vi "MFLI read data.vi"(6 "Module":T3, 7 "ModuleHandles in":T5[](array[typedef]) {"ModHandle" format="0x%08x"; "Conn" format="0x%08x"}, 8 "error in (no error)":errorcluster, 9 "lock-in handle in":T1 {"Handle" format="0x%08x"; "Conn" format="0x%08x"}, 10 "Mode":T2, 11 "Queue in":T4) -> (2 "ModuleHandles out":T5[](array[typedef]) {"ModHandle" format="0x%08x"; "Conn" format="0x%08x"}, 3 "Handle Out out":T1 {"Handle" format="0x%08x"; "Conn" format="0x%08x"})   [LabVIEW 2024, in "Lock-in module.lvlib"]
uses:
  Lock-in module.lvlib
  <instrlib>/Zurich Instruments LabOne/Public/Modules/ziTypeModHandle.ctl
  Messenger service/Data types/Mailbox address.ctl
  Messenger service/Data types/Module name.ctl
  <instrlib>/Zurich Instruments LabOne/Public/ziTypeHandle.ctl
  ctl/Mode.ctl
  <instrlib>/Zurich Instruments LabOne/Public/Modules/ziTypeModEnum.ctl
  ctl/ADQ data.ctl
  <instrlib>/Zurich Instruments LabOne/Public/Configure/ziGetValueDemodSampleEx.vi
  <instrlib>/Zurich Instruments LabOne/Public/Modules/ziModGetScopeWave.vi
  <instrlib>/Zurich Instruments LabOne/Zurich Instruments LabOne.lvlib
  Messenger service/MessengerLib.lvlib
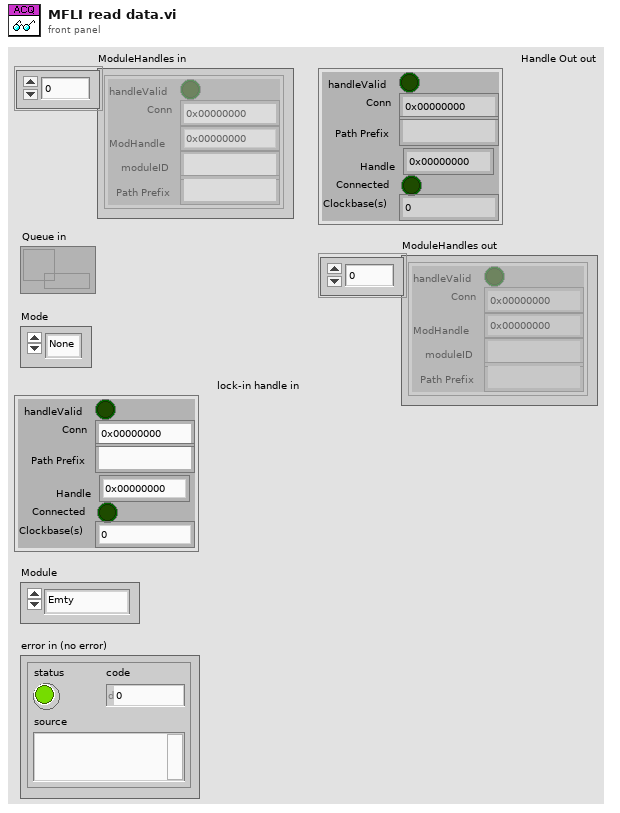
[diagram p1: front panel]
types:
  T1 = typedef "Zurich Instruments LabOne.lvlib/ziTypeHandle.ctl" = cluster{"handleValid":bool, "Conn":u64, "Path Prefix":string, "Handle":u64, "Connected":bool, "Clockbase(s)":dbl}
  T2 = typedef "Lock-in module.lvlib/Mode.ctl" = enum16{"None", "Point", "Scope", "Both", "DAQ"}
  T3 = typedef "Module name.ctl" = enum16{"Emty", "Magnet", "VTI", "Excitation", "Servo", "Acquisition", "Rotator", "Digitizer", "SMU2450", "Carousel", "Multimeter", "Tmp monitor", "Power monitor"}
  T4 = typedef "MessengerLib.lvlib/Mailbox address.ctl" = refnum<queue>
  T5 = typedef "Zurich Instruments LabOne.lvlib/ziTypeModHandle.ctl" = cluster{"handleValid":bool, "Conn":u64, "ModHandle":u64, "moduleID":string, "Path Prefix":string}
  T6 = typedef "Lock-in module.lvlib/ADQ data.ctl" = cluster{"X":sgl[], "Y":sgl[]}
  T7 = typedef "Zurich Instruments LabOne.lvlib/ziTypeDemodSampleSingle.ctl" = cluster{"Timestamps (ticks)":u64, "X (Vrms)":dbl, "Y (Vrms)":dbl, "Osc Phase (deg)":dbl, "Freq (Hz)":dbl, "DIO":u32, "AuxIn0 (V)":dbl, "AuxIn1 (V)":dbl, "Trigger":u32}
  T8 = typedef "Zurich Instruments LabOne.lvlib/ziTypeModEnum.ctl" = u16
  T9 = typedef "Zurich Instruments LabOne.lvlib/ziTypeModResults.ctl" = cluster{"PathArray":string[], "ValueType":T10, "NoOfResults":u64, "ziGenericHeader":T11[]}
  T10 = typedef "Zurich Instruments LabOne.lvlib/ziTypePollType.ctl" = enum16{"NONE", "DOUBLE_DATA", "INTEGER_DATA", "DEMOD_SAMPLE", "SCOPE_WAVE_HF2", "AUXIN_SAMPLE", "DIO_SAMPLE", "BYTE_ARRAY", "PWA_WAVE", "9", "10", "11", "12", "13", "14", "15", "TREE_CHANGE_DEPRI", "17", "ERROR", "19", "20", "21", "22", "23", "24", "25", "26", "27", "28", "29", "30", "31", "DOUBLE_DATA_TS", "INTEGER_DATA_TS", "34", "SCOPE_WAVE", "SCOPE_WAVE_EX", "37", "BYTE_ARRAY_TS", "39", "40", "41", "42", "43", "44", "45", "CNT_DATA", "47", "TREE_CHANGE", "49", "50", "51", "52", "53", "54", "55", "56", "57", "58", "59", "60", "61", "62", "63", "SWEEPER_DATA", "SPECTRUM_DATA", "ADVISOR_DATA", "VECTOR_DATA", "IMP_DATA"}
  T11 = typedef "Zurich Instruments LabOne.lvlib/ziTypeModGenericHeader.ctl" = cluster{"HeaderType":enum8{"HEADER_TYPE_NONE", "HEADER_TYPE_SWTRIGGER", "HEADER_TYPE_SWEEPER"}, "SampleFormat":u8, "SystemTime":timestamp, "CreatedTimeStamp":u64, "ChangedTimeStamp":u64, "Flags":u32, "ChunkSizeBytes":u64, "Name":string, "Status":u32, "GroupIndex":u32, "Color":u32, "ActiveRow":u32, "TriggerNumber":u64, "GridRows":u32, "GridCols":u32, "GridMode":u32, "GridOperation":u32, "GridDirection":u32, "GridRepetitions":u32, "GridColDelta":dbl, "GridColOffset":dbl, "GridRowDelta":dbl, "GridRowOffset":dbl, "Bandwidth":dbl, "Center":dbl, "Nenbw":dbl}
  T12 = typedef "Zurich Instruments LabOne.lvlib/ziTypeScopeWave.ctl" = cluster{"Timestamp (ticks)":u64, "Timestamp Trigger (ticks)":u64, "dt (s)":dbl, "Channel Enable":u8[], "Channel Input":enum8{"Signal Input 1", "Signal Input 2", "Trigger Input 1", "Trigger Input 2", "Aux Output 1", "Aux Output 2", "Aux Output 3", "Aux Output 4", "Aux Input 1", "Aux Input 2"}[], "Trigger Enable":u64, "Trigger Input":u64, "Channel BW Limit":u8[], "Channel Math":u8[], "Channel Scaling":sgl[], "Sequence Number":u32, "Segment Number":u32, "Block Number":u32, "Data Transfer Mode":enum8{"Single Transfer", "Block Transfer", "Continuous Transfer", "FFT Single Transfer"}, "Block Marker":enum8{"None", "End of Block"}, "Flags":u8, "Sample Format":enum8{"Int16", "Int32", "Float32", "reserved", "Int16 Interleaved", "Int32 Interleaved", "Float32 Interleaved"}, "Sample Count":u32, "Channel Offset":dbl[], "Data Int16":i16[], "Data Int32":i32[], "Data Float":sgl[], "Total Samples":u64}
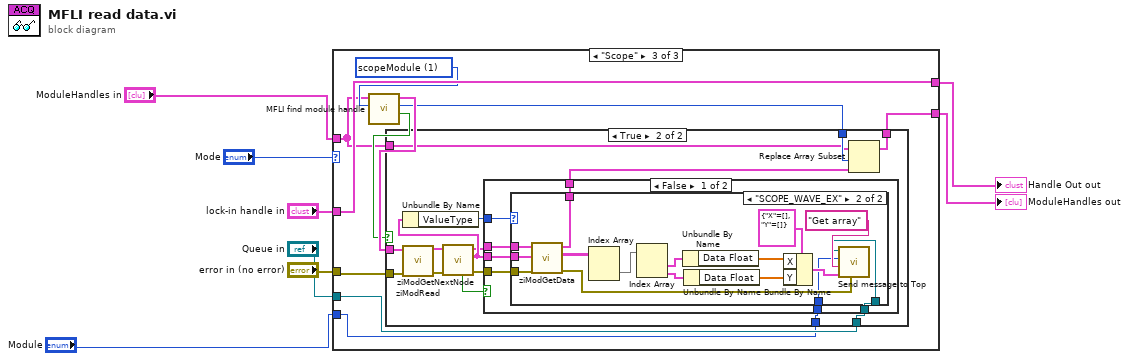
[diagram p0: block diagram]
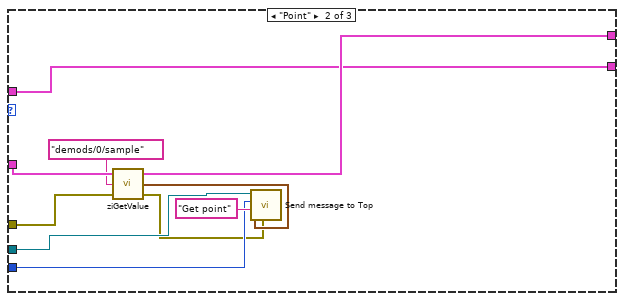
[diagram p3: hidden frame]
diagram:
  n1 = case shown="\"Scope\"" "Mode" {
    tunnel: [w10 w20 w30] -> w1
    tunnel: "lock-in handle in" -> [w10 w19 w30]
    tunnel: "Module" -> [_ w14 w27]
    tunnel: "error in (no error)" -> [_ w17 w29]
    tunnel: "Queue in" -> [_ w15 w28]
    tunnel: "ModuleHandles in" -> [w9 w11 w22]
    tunnel: [w9 w11 w21] -> w8
    frame "None", Default {
    }
    frame "Point" {
      n2 = call-poly <instrlib>:"ziGetValue.vi"("error in"=w17, "Path"="demods/0/sample", "Handle In"=w19) -> ("error out"=w12:errorcluster, "Demod Sample Out"=w13:T7, "Handle Out"=w20:T1)
      n3 = call "Send message to Top.vi"("Error in (no error)"=w12, "Data"=w13, "Response"="Get point", "Module"=w14, "Mailbox address in"=w15) -> ()  [unwired: 5 in, 2 out]
    }
    frame "Scope" {
      w26 = T8 1 items=["sweep", "scopeModule", "dataAcquisitionModule", "pidAdvisor", "awgModule", "impedanceModule", "multiDeviceSyncModule", "zoomFFT", "trigger", "deviceSettings", "record"] ("module Id")
      n4 = call "MFLI find module handle.vi"("module Id"=w26, "ModuleHandles"=w22) -> ("was found"=w24:bool, "index"=w23:i32, "ziModHandle out"=w25:T5)  [unwired: 7 in]
      n5 = case shown="True" w24 {
        tunnel: w29 -> [_ w39]
        tunnel: w28 -> [_ w38]
        tunnel: w27 -> [_ w37]
        tunnel: w25 -> [_ w36]
        tunnel: w23 -> [_ w35]
        tunnel: w22 -> [w31 w34]
        tunnel: [w31 w32] -> w21
        frame False {
        }
        frame True {
          n6 = call <instrlib>:"ziModRead.vi"("error in"=w39, "ziModHandle In"=w36) -> ("error out"=w41:errorcluster, "ziModHandle Out"=w40:T5)  [unwired: 8 in]
          n7 = call <instrlib>:"ziModGetNextNode.vi"("Error In"=w41, "ModHandle In"=w40) -> ("Error Out"=w46:errorcluster, "ModResults"=w45:T9, "ModHandle Out"=w44:T5, "NoData"=w42:bool)  [unwired: 6 in]
          n8 = Unbundle By Name(w45) -> ("ValueType"=w43:T10)
          n9 = case shown="False" w42 {
            tunnel: w43 -> [w53 _]
            tunnel: w44 -> [w52 w71]
            tunnel: w45 -> [w51 _]
            tunnel: w46 -> [w50 _]
            tunnel: [w49 w71] -> w33
            tunnel: w38 -> [w48 _]
            tunnel: w37 -> [w47 _]
            frame False {
              n10 = case shown="\"SCOPE_WAVE_EX\"" w53 {
                tunnel: w52 -> [w54 w70]
                tunnel: w51 -> [_ w69]
                tunnel: w50 -> [_ w68]
                tunnel: [w54 w57] -> w49
                tunnel: w48 -> [_ w56]
                tunnel: w47 -> [_ w55]
                frame "NONE", Default {
                }
                frame "SCOPE_WAVE_EX" {
                  n11 = call-poly <instrlib>:"ziModGetData.vi"("Error In"=w68, "ModResults"=w69, "ModHandle In"=w70) -> ("Error Out"=w58:errorcluster, "ModScopeWave"=w67:T12[][], "ModHandle Out"=w57:T5)  [unwired: 5 in, 1 out]
                  n12 = Index Array(array=w67) -> (element=w66:T12[])  [unwired: 2 in]
                  n13 = Index Array(array=w66) -> (element #1=w65:T12, element #2=w64:T12)  [unwired: 2 in]
                  n14 = Unbundle By Name(w65) -> ("Data Float"=w61:sgl[])
                  n15 = Unbundle By Name(w64) -> ("Data Float"=w60:sgl[])
                  n16 = Bundle By Name(cluster=T6 {"X"=[], "Y"=[]} ("ADQ data"), "X"=w61, "Y"=w60) -> (w59:T6)
                  n17 = call "Send message to Top.vi"("Error in (no error)"=w58, "Data"=w59, "Response"="Get array", "Module"=w55, "Mailbox address in"=w56) -> ()  [unwired: 5 in, 2 out]
                }
              }
            }
            frame True {
            }
          }
          n18 = Replace Array Subset(array=w34, new element=w33, index=w35) -> (w32:T5[])
        }
      }
    }
  }
  "ModuleHandles out" <- w8
  "Handle Out out" <- w1
